vi "XYZAER Loop Sample.vi"() -> ()   [LabVIEW 2019]
doc: "XYZAER Loop Sample demonstrates the use of the <B>XYZAER Loop VI</B>. \n\nIt displays P&O data only, in a 1-D array of <B>6VEC</B> typedefs. (<B>PDI 6VEC.ctl</B>).\n\nAlso demonstrated are <B>PDI util sensorcount.vi</B> and <B>PDI config setbuffer.vi</B>."
uses:
  Instance           3 30Saved   PDI XYZAER Loop Sample .vi
panel:
  in  "XYZAER":T1(array[cluster]) {"r" format="%1_6f"; "e" format="%1_6f"; "a" format="%1_6f"; "z" format="%1_6f"; "y" format="%1_6f"; "x" format="%1_6f"}
  in  "stop":bool
  out "Running":bool
  out "HostFrameCount":u32
  out "error out":errorcluster {"code" format="%.0x"}
  out "Elapsed Time Text":string
  out "Stop Time Text":string
  out "Start Time Text":string
  out "Loop Iter":i32
  out "PnoData":bool
  out "Connected":bool
  # "XYZAER Loop Sample demonstrates the use of the XYZAER Loop VI. \nIt displays P&O data only, in a 1-D array of 6VEC typedefs. (PDI 6VEC.ctl).\nAlso demonstrated are PDI util sensorcount.vi and PDI config setbuffer.vi."
  # "XYZAER array is an array of \"6VEC\" clusters, from the 6VEC strict typedef\nin PDI 6VEC.ctl.  In this instance the 6VEC clusters have been detached from \nthe typedef, so that they could be re-shaped to a horizontal display."
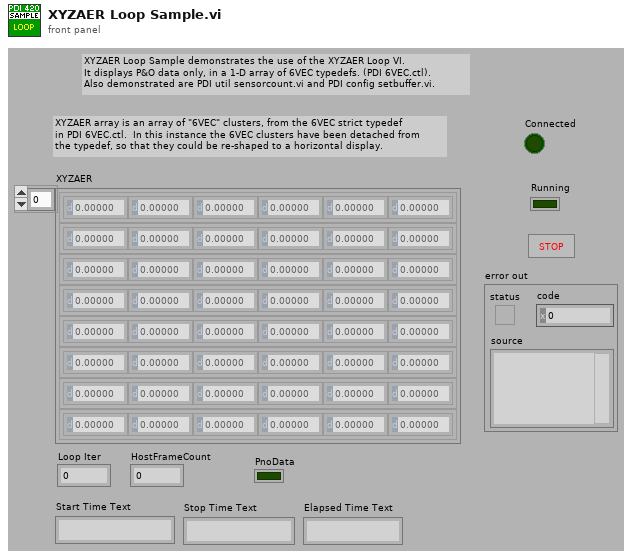
[diagram p1: front panel]
types:
  T1 = cluster{"x":sgl, "y":sgl, "z":sgl, "a":sgl, "e":sgl, "r":sgl}[]
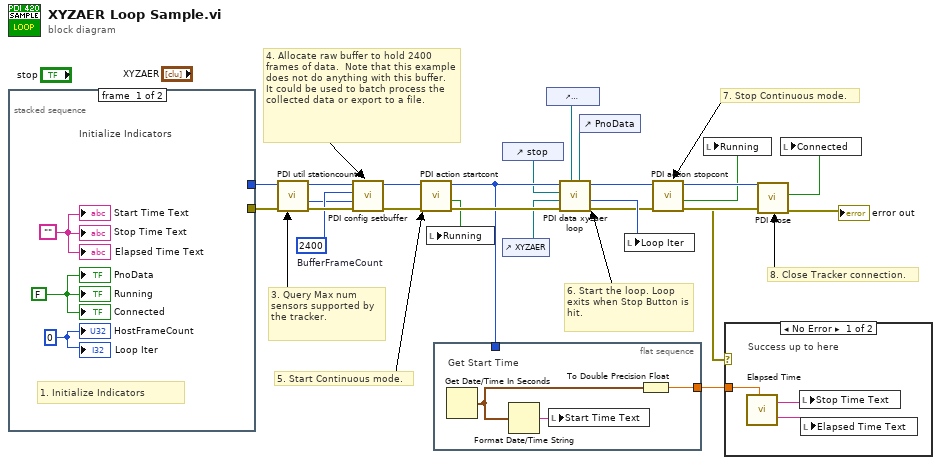
[diagram p0: block diagram]
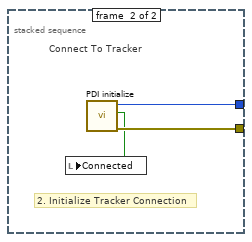
[diagram p3: hidden frame]
diagram:
  w3 = 2400  # BufferFrameCount
  # "8. Close Tracker connection."
  # "3. Query Max num sensors supported by the tracker."
  # "4. Allocate raw buffer to hold 2400 frames of data.  Note that this example does not do anything with this buffer.  It could be used to batch process the collected data or export to a file."
  # "5. Start Continuous mode."
  # "7. Stop Continuous mode."
  # "6. Start the loop. Loop exits when Stop Button is hit."
  n1 = stacked-sequence {
    tunnel: [_ w30] -> w7
    tunnel: [_ w29] -> w6
    frame #0 {
      w25 = 0
      w26 = FALSE
      w27 = ""
      # "Initialize Indicators"
      # "1. Initialize Indicators"
      "Connected" <- w26
      "Start Time Text" <- w27
      "Stop Time Text" <- w27
      "Elapsed Time Text" <- w27
      "HostFrameCount" <- w25
      "Running" <- w26
      "Loop Iter" <- w25
      "PnoData" <- w26
    }
    frame #1 {
      # "Connect To Tracker"
      # "2. Initialize Tracker Connection"
      n2 = call <instrlib>:"PDI initialize.vi"() -> ("error out"=w29:errorcluster, "Connected"=w28:bool, "pDev"=w30:u32)  [unwired: 1 in, 4 out]
      n3 = local write "Connected"(w28) -> ()
    }
  }
  n4 = call <instrlib>:"PDI util stationcount.vi"("error in (no error)"=w6, "pDev"=w7) -> ("error out"=w5:errorcluster, "dup pDev"=w4:u32, "MaxCount"=w2:i32)  [unwired: 7 out]
  n5 = call <instrlib>:"PDI config setbuffer.vi"("error in (no error)"=w5, "Max sensors"=w2, "FrameCount"=w3, "pDev"=w4) -> ("error out"=w14:errorcluster, "dup pDev"=w15:u32)  [unwired: 6 out]
  n6 = call <instrlib>:"PDI action startcont.vi"("error in (no error)"=w14, "pDev"=w15) -> ("error out"=w21:errorcluster, "Running"=w13:bool, "dup pDev"=w20:u32)  [unwired: 7 out]
  n7 = local write "Running"(w13) -> ()
  n8 = flat-sequence {
    tunnel: w20 -> [_]
    tunnel: [w31] -> w16
    frame #0 {
      # "Get Start Time"
      n9 = Get Date/Time In Seconds() -> (seconds since 1Jan1904=w32:timestamp)
      n10 = Format Date/Time String(seconds (now)=w32) -> (date/time string=w33:string)  [unwired: 2 out]
      n11 = local write "Start Time Text"(w33) -> ()
      n12 = To Double Precision Float(number=w32) -> (double precision float=w31:dbl)
    }
  }
  n13 = control-ref of="stop"() -> (w19:refnum<vi>)
  n14 = control-ref of="XYZAER"() -> (w10:refnum<vi>)
  n15 = control-ref of="HostFrameCount"() -> (w11:refnum<vi>)
  n16 = control-ref of="PnoData"() -> (w1:refnum<vi>)
  n17 = call <instrlib>:"PDI data xyzaer loop.vi"("Data Ready Refnum"=w1, "FrameCount Ctl Ref"=w11, "error in (no error)"=w21, "xyzaer array\nRefnum"=w10, "Stop Ctl Ref"=w19, "pDev"=w20) -> ("error out"=w8:errorcluster, "Loop Iter"=w12:i32, "dup pDev"=w9:u32)  [unwired: 3 out]
  n18 = local write "Loop Iter"(w12) -> ()
  n19 = call <instrlib>:"PDI action stopcont.vi"("error in (no error)"=w8, "pDev"=w9) -> ("error out"=w17:errorcluster, "Running"=w22:bool, "dup pDev"=w23:u32)  [unwired: 7 out]
  n20 = local write "Running"(w22) -> ()
  n21 = case shown="No Error" w8 {
    tunnel: w16 -> [w34 _]
    frame No Error {
      # "Success up to here"
      n22 = call "Elapsed Time"("Set Start Time (s)"=w34) -> ("Present Text"=w36:string, "Elapsed Time Text"=w35:string)  [unwired: 4 in, 13 out]
      n23 = local write "Stop Time Text"(w36) -> ()
      n24 = local write "Elapsed Time Text"(w35) -> ()
    }
    frame Error {
      # "Error somewhere;\nStop Time is irrelevant"
    }
  }
  n25 = call <instrlib>:"PDI close.vi"("error in (no error)"=w17, "pDev"=w23) -> ("error out"=→"error out":errorcluster, "connected"=w18:bool)  [unwired: 8 out]
  n26 = local write "Connected"(w18) -> ()
